vi "Get Images16.vi"(5 "validlast":i32, 6 "validfirst":i32, 7 "size":u32, 9 "arr":u16, 10 "last":i32, 11 "first":i32) -> (1 "arr out":u16, 2 "function return":u32, 3 "validlast out":i32, 4 "validfirst out":i32)   [LabVIEW 2018, in "AndorSDK.lvlib"]
doc: "EXPNETTYPE unsigned int WINAPI GetImages16(long first, long last, WORD * arr, unsigned long size, long * validfirst, long * validlast);"
uses:
  AndorSDK.lvlib
  ATMCD32D.dll
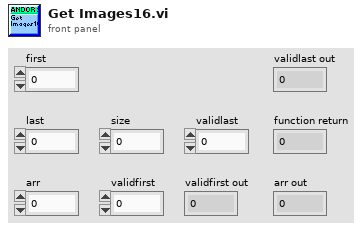
[diagram p1: front panel]
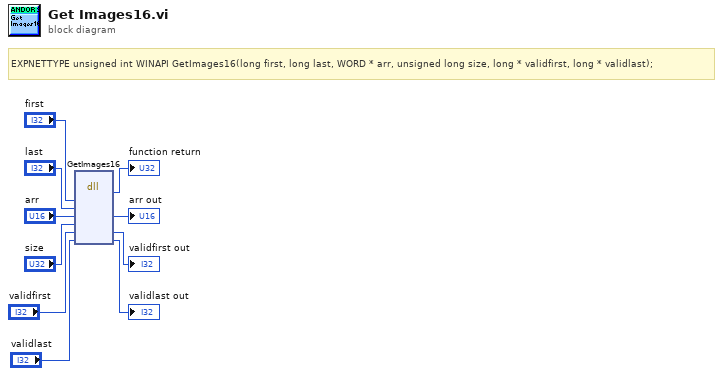
[diagram p0: block diagram]
diagram:
  # "EXPNETTYPE unsigned int WINAPI GetImages16(long first, long last, WORD * arr, unsigned long size, long * validfirst, long * validlast);"
  n1 = dll-call lib="PTH2babs E\nPersönliches02 - Arbeit03-HiwijobsLabviewCodelibANDOR\tAndor SDK\nATMCD32D.*" fn="GetImages16"("first"="first", "last"="last", "arr"="arr", "size"="size", "validfirst"="validfirst", "validlast"="validlast") -> (→"function return":u32, "arr"=→"arr out":u16, "validfirst"=→"validfirst out":i32, "validlast"=→"validlast out":i32)  [unwired: 6 in, 2 out]
